vi "gpibtalk_JHC.vi"(2 "error in":errorcluster, 3 "milliseconds to wait (10)":u32=10, 4 "Send":string, 5 "Inst (F:Temp T:Res)":bool=TRUE) -> (0 "error out":errorcluster, 1 "read":string="\n")   [LabVIEW 2013]
panel:
  # "RESISTANCE"
  # "TEMPERATURE"
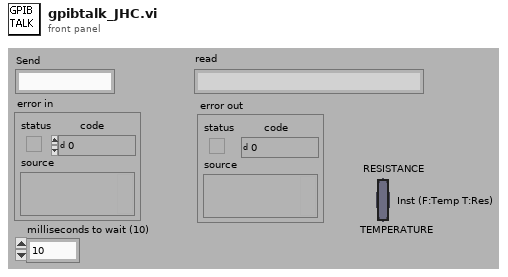
[diagram p1: front panel]
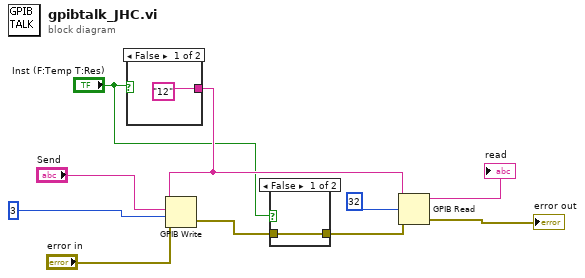
[diagram p0: block diagram]
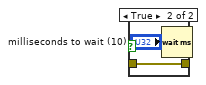
[diagram p2: hidden frame]
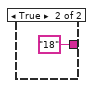
[diagram p3: hidden frame]
diagram:
  n1 = case shown="False" "Inst (F:Temp T:Res)" {
    tunnel: ["12" "18"] -> w4
    frame False {
    }
    frame True {
    }
  }
  n2 = GPIB Write(0:w4, 1:"Send", 2:i16 3 ("mode (0)"), 3:"error in") -> (6:w9:errorcluster)  [unwired: 1 in, 1 out]
  n3 = case shown="False" "Inst (F:Temp T:Res)" {
    tunnel: w9 -> [w13 w15]
    tunnel: [w13 w15] -> w10
    frame False {
    }
    frame True {
      n4 = Wait (ms)(milliseconds to wait="milliseconds to wait (10)") -> ()  [unwired: 1 out]
    }
  }
  n5 = GPIB Read(0:w4, 1:i16 32 ("mode (0)"), 3:w10) -> (5:→"read":string, 7:→"error out":errorcluster)  [unwired: 2 in, 1 out]
